vi "KeythleyDMM6500_04582450.vi"(4 "error in":T14, 7 "Command":T15) -> (0 "error out":T14, 3 "Response":T12)   [LabVIEW 2018]
uses:
  MOKO_LabViewLibrary/MokoLowLevel/MokoLowLovelControl/MLLC_Command.ctl
  MOKO_LabViewLibrary/MokoLowLevel/MokoLowLovelControl/MLLC_Error.ctl
  MOKO_LabViewLibrary/MokoLowLevel/MokoLowLovelControl/MLLC_Mode.ctl
  MOKO_LabViewLibrary/MokoLowLevel/MokoLowLovelControl/MLLC_Response.ctl
  MOKO_LabViewLibrary/MokoLowLevel/MokoLowLovelControl/MLLC_DriverName.ctl
  MOKO_LabViewLibrary/MokoLowLevel/MokoLowLovelControl/MLLC_Request.ctl
  MOKO_LabViewLibrary/MokoLowLevel/MokoLowLovelControl/MLLC_ErrorCode.ctl
  MOKO_LabViewLibrary/MokoLowLevel/MokoLowLovelControl/MLLC_ResponseInit.ctl
  MOKO_LabViewLibrary/MokoLowLevel/MokoLowLovelControl/MLLC_ConnectCluster.ctl
  MOKO_LabViewLibrary/MokoLowLevel/MokoLowLovelControl/MLLC_InterfaceType.ctl
  MOKO_LabViewLibrary/MokoLowLevel/MokoLowLovelControl/MLLC_OpenedSession.ctl
  MOKO_LabViewLibrary/MokoLowLevel/MokoLowLovelControl/MLLC_InterfaceSettings.ctl
  MOKO_LabViewLibrary/MokoLowLevel/MokoLowLovelControl/MLLC_InterfaceKind.ctl
  data/KeythleyDMM6500_Functions.ctl
panel:
  in  "Settings":T8={"Saved Data"=variant, "Data"={"Connect"={"InterfaceType"=enum."VISA", "OpenedSession"="", "InterfaceSettings"={"Interface"=enum."GPIB", "EOS 4 read"=enum."LF (\\n)", "EOS 4 write"=enum."LF (\\n)", "TMO, ms"=5000, "Sett"=variant(cluster{"Baud Rate":u32, "Data Bits":u16, "Parity":u16, "Stop Bits":u16, "Flow Control":u16, "Eho":bool} {"Baud Rate"=75, "Data Bits"=0, "Parity"=0, "Stop Bits"=0, "Flow Control"=0, "Eho"=FALSE})}}, "Channel"=1, "Func"=enum."IDC"}}
  in  "Response Init array":T9="DMM6500,04582450"
  in  "Error Code":T6=5475
  in  "Request":T10="*idn?"
  in  "Driver Name":T11="DMM6500_04582450"
  in  "Mode":T13=enum."Check"
  # "KEITHLEY INSTRUMENTS,MODEL DMM6500,04582450,1.7.12b = U"
  # "KEITHLEY INSTRUMENTS,MODEL DMM6500,04625545,1.7.12b = I"
  # "KeythleyDMM6500_04582450"
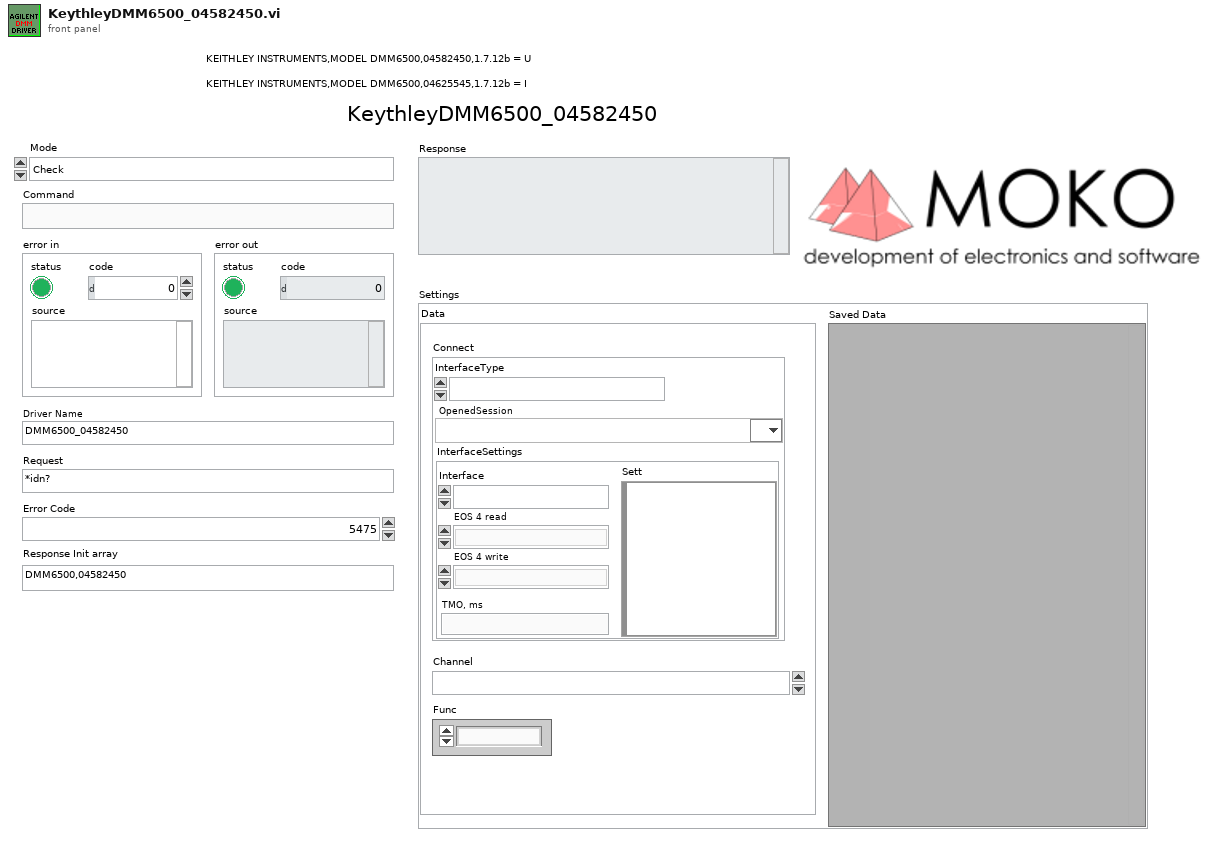
[diagram p1: front panel]
types:
  T1 = typedef "MLLC_ConnectCluster.ctl" = cluster{"InterfaceType":T2, "OpenedSession":T3, "InterfaceSettings":T4}
  T2 = typedef "MLLC_InterfaceType.ctl" = enum16{"VISA", "Prologix USB-GPIB"}
  T3 = typedef "MLLC_OpenedSession.ctl" = refnum<visa-resource-name>
  T4 = typedef "MLLC_InterfaceSettings.ctl" = cluster{"Interface":T5, "EOS 4 read":enum16{"Default (=EOS 4 write)", "CR (\\r)", "LF (\\n)", "None"}, "EOS 4 write":enum16{"CR+LF (\\r\\n)", "CR (\\r)", "LF (\\n)", "None"}, "TMO, ms":i32, "Sett":variant}
  T5 = typedef "MLLC_InterfaceKind.ctl" = enum16{"RS232", "GPIB", "USB", "Ethernet", "another"}
  T6 = typedef "MLLC_ErrorCode.ctl" = u32
  T7 = typedef "KeythleyDMM6500_Functions.ctl" = enum16{"VDC", "VAC", "IDC", "IAC", "F", "R2", "R4", "CAP"}
  T8 = cluster{"Saved Data":variant, "Data":cluster{"Connect":T1, "Channel":T6, "Func":T7}}
  T9 = typedef "MLLC_ResponseInit.ctl" = string
  T10 = typedef "MLLC_Request.ctl" = string
  T11 = typedef "MLLC_DriverName.ctl" = string
  T12 = typedef "MLLC_Response.ctl" = string
  T13 = typedef "MLLC_Mode.ctl" = enum16{"get", "set", "close", "Init", "Check"}
  T14 = typedef "MLLC_Error.ctl" = errorcluster
  T15 = typedef "MLLC_Command.ctl" = string
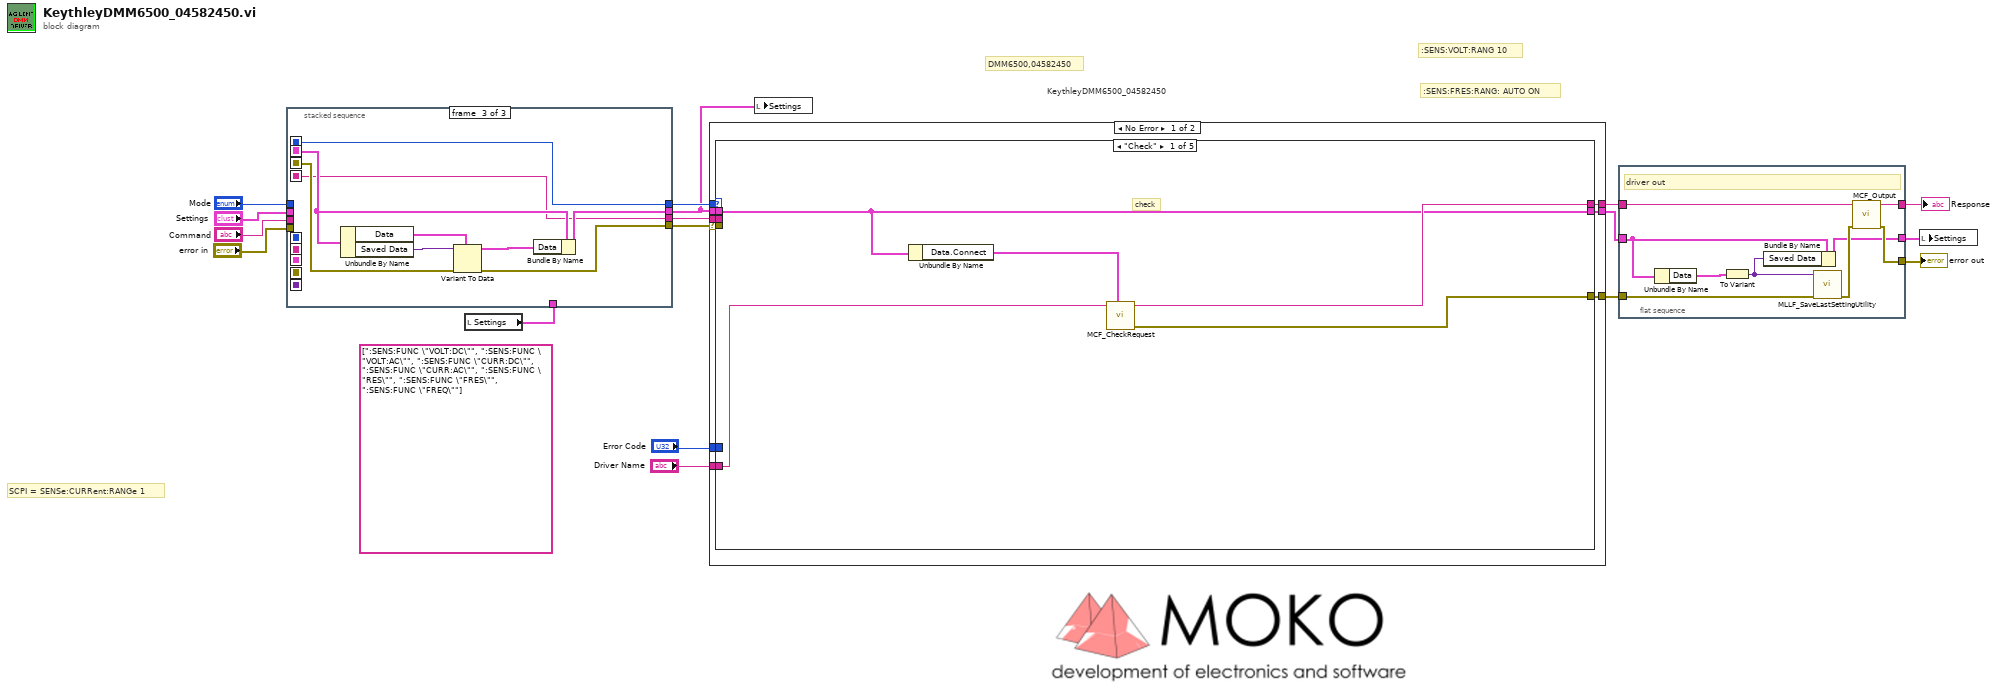
[diagram p0: block diagram]
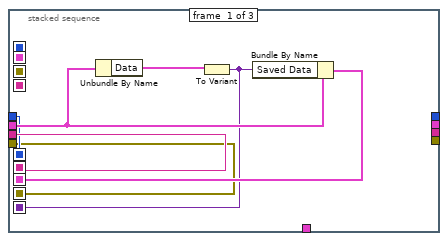
[diagram p2: hidden frame]
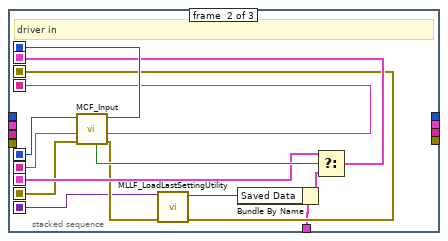
[diagram p3: hidden frame]
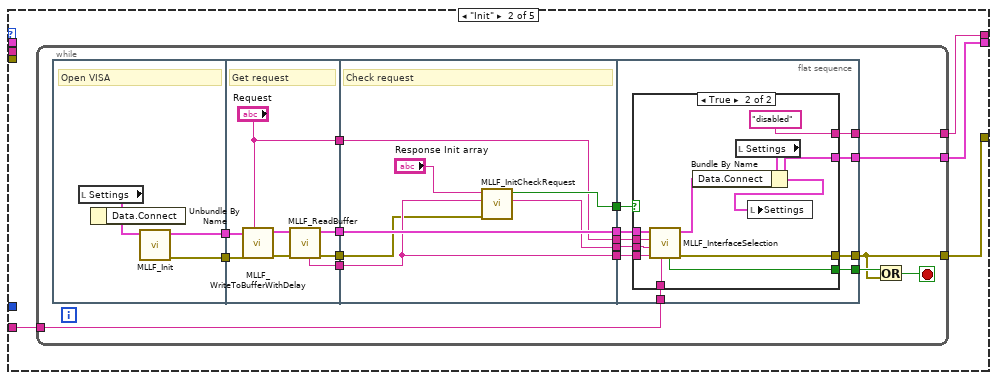
[diagram p4: hidden frame]
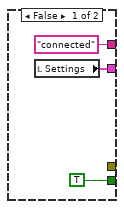
[diagram p5: hidden frame]
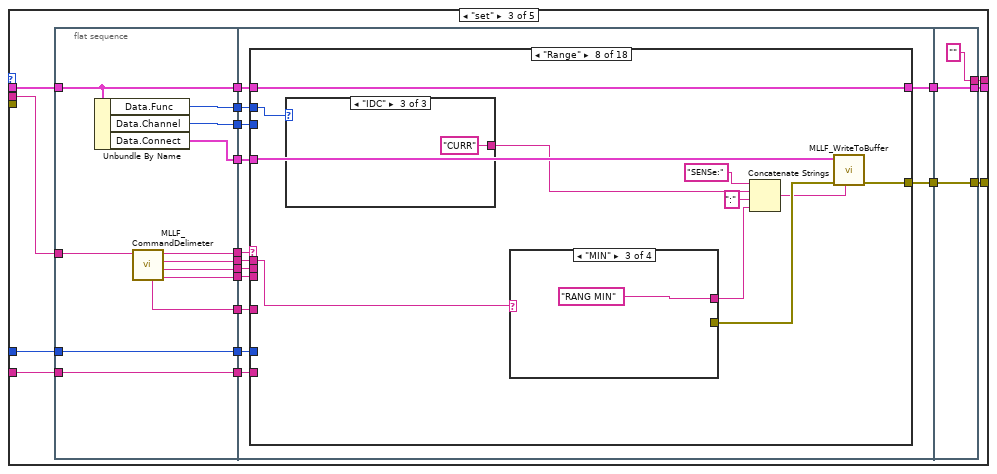
[diagram p6: hidden frame]
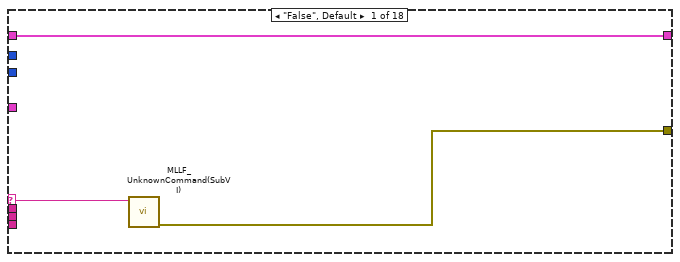
[diagram p7: hidden frame]
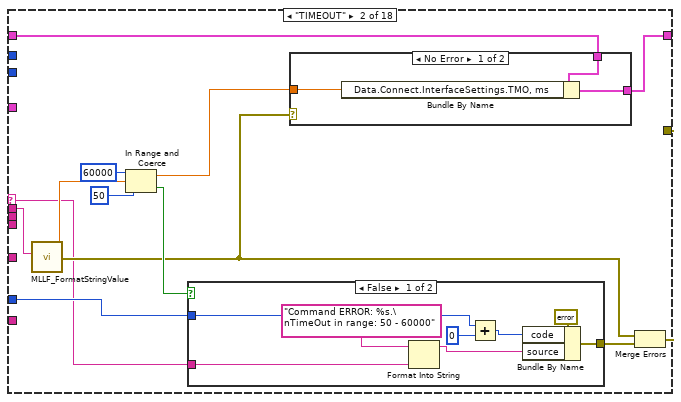
[diagram p8: hidden frame]
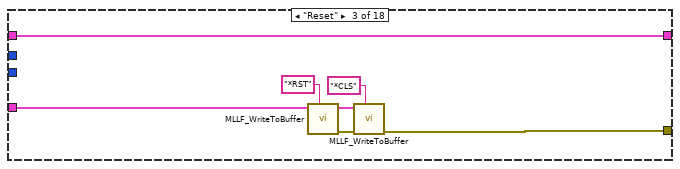
[diagram p11: hidden frame]
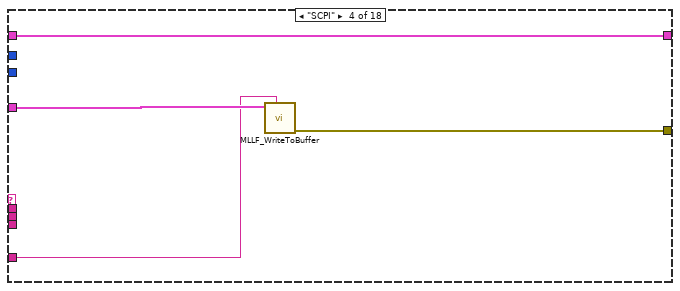
[diagram p12: hidden frame]
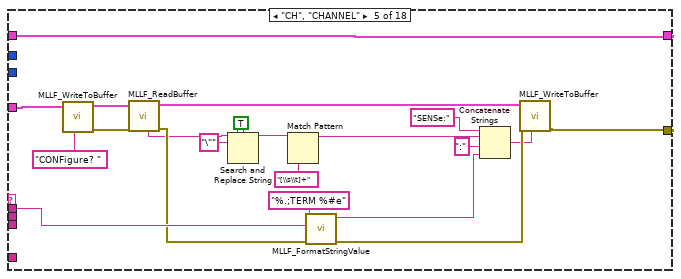
[diagram p13: hidden frame]
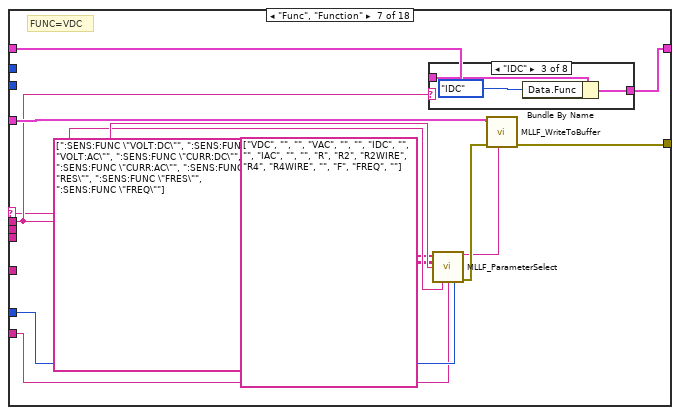
[diagram p15: hidden frame]
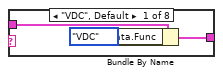
[diagram p16: hidden frame]
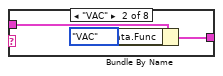
[diagram p17: hidden frame]
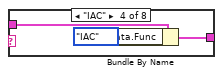
[diagram p18: hidden frame]
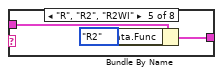
[diagram p19: hidden frame]
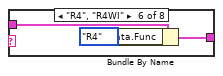
[diagram p20: hidden frame]
diagram:
  (unwired) string[] [":SENS:FUNC \"VOLT:DC\"", ":SENS:FUNC \"VOLT:AC\"", ":SENS:FUNC \"CURR:DC\"", ":SENS:FUNC \"CURR:AC\"", ":SENS:FUNC \"RES\"", ":SENS:FUNC \"FRES\"", ":SENS:FUNC \"FREQ\""] ("Names")
  # ":SENS:FRES:RANG: AUTO ON"
  # ":SENS:VOLT:RANG 10"
  # "DMM6500,04582450"
  # "SCPI = SENSe:CURRent:RANGe 1"
  # "KeythleyDMM6500_04582450"
  n1 = local read "Settings"() -> (w8:T8)
  n2 = stacked-sequence {
    seq-local: [w20 _ _] -> [_ w36 _]
    seq-local: [w19 _ _] -> [_ w37 _]
    seq-local: [w22 _ _] -> [_ w32 _]
    seq-local: [w18 _ _] -> [_ w31 _]
    seq-local: [w21 _ _] -> [_ w27 _]
    seq-local: [_ w28 _] -> [_ _ w44]
    seq-local: [_ w38 _] -> [_ _ w41]
    seq-local: [_ w35 _] -> [_ _ w40]
    seq-local: [_ w34 _] -> [_ _ w45]
    tunnel: "Command" -> [w20 _ _]
    tunnel: "Mode" -> [w19 _ _]
    tunnel: "error in" -> [w18 _ _]
    tunnel: "Settings" -> [w23 _ _]
    tunnel: w8 -> [_ w26 _]
    tunnel: [_ _ w40] -> w10
    tunnel: [_ _ w43] -> w2
    tunnel: [_ _ w42] -> w9
    tunnel: [_ _ w41] -> w11
    frame #0 {
      n3 = Unbundle By Name(w23) -> ("Data"=w24:cluster{"Connect":T1, "Channel":T6, "Func":T7})
      n4 = To Variant(anything=w24) -> (Variant=w21:variant)
      n5 = Bundle By Name(cluster=w23, "Saved Data"=w21) -> (w22:T8)
    }
    frame #1 {
      # "driver in"
      n6 = call "MCF_Input.vi"("Error In"=w31, "Command in"=w36, "Mode in"=w37) -> ("Error Out"=w30:errorcluster, "Command out"=w35:string, "Mode out"=w38:T13, "Boolean"=w33:bool)  [unwired: 5 in]
      n7 = call "MLLF_LoadLastSettingUtility.vi"("Error In"=w30, "Save data in"=w27) -> ("Error Out"=w28:errorcluster, "Save data out"=w25:variant)  [unwired: 8 in]
      n8 = Bundle By Name(cluster=w26, "Saved Data"=w25) -> (w29:T8)
      n9 = Select(t=w32, s=w33, f=w29) -> (s? t:f=w34:T8)
    }
    frame #2 {
      n10 = Unbundle By Name(w45) -> ("Data"=w46:cluster{"Connect":T1, "Channel":T6, "Func":T7}, "Saved Data"=w39:variant)
      n11 = Variant To Data(error in=w44, type=w46, Variant=w39) -> (data=w47:cluster{"Connect":T1, "Channel":T6, "Func":T7}, error out=w42:errorcluster)
      n12 = Bundle By Name(cluster=w45, "Data"=w47) -> (w43:T8)
    }
  }
  n13 = case shown="No Error" w9 {
    selector: w9 -> [w53 w582]
    tunnel: [w54 w582] -> w5
    tunnel: w11 -> [w56 _]
    tunnel: [w55 "An error occurred in the driver input module." ("String")] -> w7
    tunnel: w10 -> [w48 _]
    tunnel: w2 -> [w49 w581]
    tunnel: "Error Code" -> [w52 _]
    tunnel: "Driver Name" -> [w51 _]
    tunnel: [w50 w581] -> w6
    frame No Error {
      n14 = case shown="\"Check\"" w56 {
        tunnel: [w60 w65 w139 w508 "" ("String")] -> w55
        tunnel: [w61 w63 w142 w509 w578] -> w54
        tunnel: w53 -> [_ _ _ w523 _]
        tunnel: w52 -> [_ _ w145 w525 _]
        tunnel: w51 -> [w59 w62 w143 w524 _]
        tunnel: [w57 w64 w144 w526 w577] -> w50
        tunnel: w49 -> [w57 _ w128 w514 w577]
        tunnel: w48 -> [_ _ w127 w513 _]
        frame "Check" {
          # "check"
          n15 = Unbundle By Name(w57) -> ("Data.Connect"=w58:T1)
          n16 = call "MCF_CheckRequest.vi"("Permanent data.Connect"=w58, "Driver Name"=w59) -> ("Error Out"=w61:errorcluster, "Output String"=w60:string)  [unwired: 8 in]
        }
        frame "Init" {
          n17 = while {
            tunnel: [w71] -> w63
            tunnel: [w70] -> w65
            tunnel: [w69] -> w64
            tunnel: w62 -> [w73]
            stop <- w82 stop-if-true
            n18 = flat-sequence {
              tunnel: [w86] -> w81
              tunnel: [w85] -> w80
              tunnel: w81 -> [w92]
              tunnel: w80 -> [w91]
              tunnel: [w90] -> w79
              tunnel: [w89] -> w78
              tunnel: [w88] -> w77
              tunnel: ["Request"] -> w67
              tunnel: w79 -> [w98]
              tunnel: w78 -> [w101]
              tunnel: w77 -> [w100]
              tunnel: [w101] -> w76
              tunnel: [w100] -> w75
              tunnel: [w97] -> w74
              tunnel: [w96] -> w68
              tunnel: w67 -> [w95]
              tunnel: [w95] -> w66
              tunnel: w76 -> [w110]
              tunnel: w75 -> [w109]
              tunnel: w74 -> [w111]
              tunnel: w73 -> [w108]
              tunnel: [w107] -> w72
              tunnel: [w106] -> w71
              tunnel: [w105] -> w70
              tunnel: [w104] -> w69
              tunnel: w68 -> [w103]
              tunnel: w66 -> [w102]
              frame #0 {
                # "Open VISA"
                n19 = local read "Settings"() -> (w84:T8)
                n20 = Unbundle By Name(w84) -> ("Data.Connect"=w83:T1)
                n21 = call "MLLF_Init.vi"("DriverConnect in"=w83) -> ("Error Out"=w86:errorcluster, "DriverConnect out"=w85:T1)  [unwired: 7 in]
              }
              frame #1 {
                # "Get request"
                n22 = call "MLLF_WriteToBufferWithDelay.vi"("Command"="Request", "Error In"=w92, "DriverConnect in"=w91) -> ("Error Out"=w93:errorcluster, "DriverConnect out"=w94:T1)  [unwired: 7 in]
                n23 = call "MLLF_ReadBuffer.vi"("Error In"=w93, "DriverConnect in"=w94) -> ("Error Out"=w90:errorcluster, "DriverConnect out"=w89:T1, "String"=w88:string)  [unwired: 6 in]
              }
              frame #2 {
                # "Check request"
                n24 = call "MLLF_InitCheckRequest.vi"("error in (no error)"=w98, "Answer"=w100, "Response Init"="Response Init array") -> ("ResponseInit out"=w96:string, "Design"=w97:bool)  [unwired: 5 in, 2 out]
              }
              frame #3 {
                n25 = case shown="True" w111 {
                  tunnel: w110 -> [_ w124]
                  tunnel: [TRUE w119] -> w107
                  tunnel: [_ w122] -> w106
                  tunnel: ["connected" "disabled"] -> w105
                  tunnel: [w112 w120] -> w104
                  tunnel: w109 -> [_ w117]
                  tunnel: w108 -> [_ w118]
                  tunnel: w103 -> [_ w116]
                  tunnel: w102 -> [_ w115]
                  frame False {
                    n26 = local read "Settings"() -> (w112:T8)
                  }
                  frame True {
                    n27 = call "MLLF_InterfaceSelection.vi"("Driver Name"=w118, "Answer:"=w117, "Response"=w116, "Request"=w115, "DriverConnect in"=w124) -> ("error out"=w122:T14, "DriverConnect out"=w123:T1, "stop init?"=w119:bool)  [unwired: 2 in, 2 out]
                    n28 = local read "Settings"() -> (w125:T8)
                    n29 = Bundle By Name(cluster=w125, "Data.Connect"=w123) -> (w120:T8)
                    n30 = local write "Settings"(w120) -> ()
                  }
                }
              }
            }
            n31 = Or(x=w72, y=w71) -> (x .or. y?=w82:bool)
          }
        }
        frame "set" {
          n32 = flat-sequence {
            tunnel: w143 -> [w156]
            tunnel: w128 -> [w147]
            tunnel: w145 -> [w157]
            tunnel: [w157] -> w138
            tunnel: [w147] -> w137
            tunnel: [w156] -> w136
            tunnel: [w153] -> w135
            tunnel: [w154] -> w134
            tunnel: [w155] -> w133
            tunnel: [w148] -> w132
            tunnel: [w149] -> w131
            tunnel: [w150] -> w130
            tunnel: [w151] -> w129
            tunnel: w127 -> [w152]
            tunnel: [w146] -> w126
            tunnel: [w168] -> w141
            tunnel: [w161] -> w140
            tunnel: w138 -> [w170]
            tunnel: w137 -> [w169]
            tunnel: w136 -> [w167]
            tunnel: w135 -> [w166]
            tunnel: w134 -> [w165]
            tunnel: w133 -> [w164]
            tunnel: w132 -> [w163]
            tunnel: w131 -> [w162]
            tunnel: w130 -> [w160]
            tunnel: w129 -> [w159]
            tunnel: w126 -> [w158]
            tunnel: [w506] -> w142
            tunnel: [w507] -> w144
            tunnel: w141 -> [w507]
            tunnel: w140 -> [w506]
            tunnel: ["" ("String")] -> w139
            frame #0 {
              n33 = Unbundle By Name(w147) -> ("Data.Func"=w155:T7, "Data.Channel"=w154:T6, "Data.Connect"=w153:T1)
              n34 = call "MLLF_CommandDelimeter.vi"("command with param"=w152) -> ("param 3"=w151:string, "param 2"=w150:string, "param 1"=w149:string, "command"=w148:string, "Spit delimetre"=w146:string)  [unwired: 6 in]
            }
            frame #1 {
              n35 = case shown="\"Range\"" w163 {
                selector: w163 -> [w172 w175 _ _ _ _ w237 _ _ _ _ _ _ w429 w436 w460 w484 w495]
                tunnel: w162 -> [_ w174 _ _ w228 _ w238 w277 _ w307 w320 w361 w391 w430 w437 w461 w485 w496]
                tunnel: [w171 w180 w199 w207 w210 _ w232 w271 _ w290 w319 w345 w376 w409 w435 w459 w483 w494] -> w161
                tunnel: w170 -> [_ w181 _ _ _ _ w243 _ _ _ _ _ _ w431 w441 w465 w489 w503]
                tunnel: w169 -> [w173 w185 w205 w209 w229 w231 w240 w278 w289 w309 w336 w363 w393 w434 w458 w482 w493 w504]
                tunnel: [w173 w186 w205 w209 w229 w231 w239 w278 w289 w309 w336 w363 w393 w434 w458 w482 w493 w504] -> w168
                tunnel: w166 -> [_ _ w200 w208 w230 _ w241 w269 _ w308 w335 w362 w392 w433 w457 w481 w487 w500]
                tunnel: w167 -> [_ _ _ _ _ _ w242 _ _ _ _ _ _ w432 w442 w466 w490 w502]
                tunnel: w165 -> [_ _ _ _ _ _ _ _ _ _ _ _ _ _ _ _ _ _]
                tunnel: w164 -> [_ _ _ _ _ _ _ w270 _ _ _ _ _ _ _ _ _ _]
                tunnel: w160 -> [_ _ _ _ _ _ _ _ _ _ _ _ _ _ _ _ _ _]
                tunnel: w159 -> [_ _ _ _ _ _ _ _ _ _ _ _ _ _ _ _ _ _]
                tunnel: w158 -> [_ _ _ w206 _ _ _ _ _ _ _ _ _ _ _ _ _ _]
                frame "False", Default {
                  n36 = call "MLLF_UnknownCommand(SubVI).vi"("Unknown command"=w172) -> ("error out"=w171:errorcluster)  [unwired: 10 in]
                }
                frame "TIMEOUT" {
                  n37 = call "MLLF_FormatStringValue.vi"("String Value"=w174) -> ("error out"=w176:T14, "number"=w177:dbl)  [unwired: 8 in, 1 out]
                  n38 = In Range and Coerce(upper limit=60000, x=w177, lower limit=50) -> (coerced(x)=w182:dbl, In Range?=w178:bool)
                  n39 = case shown="False" w178 {
                    tunnel: [w193 _] -> w179
                    tunnel: w181 -> [w192 _]
                    tunnel: w175 -> [w191 _]
                    frame False {
                      n40 = Format Into String(format string="Command ERROR: %s.\nTimeOut in range: 50 - 60000", w191) -> (resulting string=w195:string)  [unwired: 2 in, 1 out]
                      n41 = Add(x=w192, y=0) -> (x+y=w196:T6)
                      n42 = Bundle By Name(cluster=errorcluster {"status"=TRUE, "code"=0, "source"=""} ("error out"), "code"=w196, "source"=w195) -> (w193:errorcluster)
                    }
                    frame True {
                    }
                  }
                  n43 = case shown="No Error" w176 {
                    tunnel: [w189 w190] -> w186
                    tunnel: w185 -> [w188 w190]
                    tunnel: w182 -> [w187 _]
                    frame No Error {
                      n44 = Bundle By Name(cluster=w188, "Data.Connect.InterfaceSettings.TMO, ms"=w187) -> (w189:T8)
                    }
                    frame Error {
                    }
                  }
                  n45 = Merge Errors(w176, w179) -> (w180:errorcluster)
                }
                frame "Reset" {
                  n46 = call "MLLF_WriteToBuffer.vi"("String"="*RST", "DriverConnect in"=w200) -> ("error out"=w203:T14, "DriverConnect out"=w204:T1)  [unwired: 6 in]
                  n47 = call "MLLF_WriteToBuffer.vi"("String"="*CLS" ("write buffer"), "error in"=w203, "DriverConnect in"=w204) -> ("error out"=w199:T14)  [unwired: 5 in, 1 out]
                }
                frame "SCPI" {
                  n48 = call "MLLF_WriteToBuffer.vi"("String"=w206, "DriverConnect in"=w208) -> ("error out"=w207:T14)  [unwired: 6 in, 1 out]
                }
                frame "CH", "CHANNEL" {
                  w215 = TRUE ("replace all? (F)")
                  n49 = call "MLLF_WriteToBuffer.vi"("String"="CONFigure? ", "DriverConnect in"=w230) -> ("error out"=w224:T14, "DriverConnect out"=w225:T1)  [unwired: 6 in]
                  n50 = call "MLLF_ReadBuffer.vi"("Error In"=w224, "DriverConnect in"=w225) -> ("Error Out"=w223:errorcluster, "DriverConnect out"=w222:T1, "String"=w217:string)  [unwired: 6 in]
                  n51 = Search and Replace String(replace all?=w215, case sensitive?=w215, input string=w217, search string="\"") -> (result string=w216:string)  [unwired: 4 in, 3 out]
                  n52 = Match Pattern(string=w216, regular expression="[\\s\\t]+") -> (before substring=w218:string)  [unwired: 1 in, 3 out]
                  n53 = call "MLLF_FormatStringValue.vi"("error in"=w223, "String Value"=w228, "Format"="%.;TERM %#e" ("format string")) -> ("error out"=w227:T14, "String Value Formated"=w220:T15)  [unwired: 6 in, 1 out]
                  n54 = Concatenate Strings("SENSe:" ("string"), w218, ":" ("string"), w220) -> (w213:string)
                  n55 = call "MLLF_WriteToBuffer.vi"("String"=w213, "error in"=w227, "DriverConnect in"=w222) -> ("error out"=w210:T14)  [unwired: 5 in, 1 out]
                }
                frame "<----MAIN FUNCTIONS---->" {
                }
                frame "Func", "Function" {
                  # "FUNC=VDC"
                  n56 = case shown="\"IDC\"" w238 {
                    tunnel: w240 -> [w246 w249 w252 w255 w258 w261 w264 w267]
                    tunnel: [w245 w248 w251 w254 w257 w260 w263 w266] -> w239
                    frame "VDC", Default {
                      n57 = Bundle By Name(cluster=w246, "Data.Func"=KeythleyDMM6500_Functions."VDC" ("Func")) -> (w245:T8)
                    }
                    frame "VAC" {
                      n58 = Bundle By Name(cluster=w249, "Data.Func"=KeythleyDMM6500_Functions."VAC" ("Func")) -> (w248:T8)
                    }
                    frame "IDC" {
                      n59 = Bundle By Name(cluster=w252, "Data.Func"=KeythleyDMM6500_Functions."IDC" ("Func")) -> (w251:T8)
                    }
                    frame "IAC" {
                      n60 = Bundle By Name(cluster=w255, "Data.Func"=KeythleyDMM6500_Functions."IAC" ("Func")) -> (w254:T8)
                    }
                    frame "R", "R2", "R2WI" {
                      n61 = Bundle By Name(cluster=w258, "Data.Func"=KeythleyDMM6500_Functions."R2" ("Func")) -> (w257:T8)
                    }
                    frame "R4", "R4WI" {
                      n62 = Bundle By Name(cluster=w261, "Data.Func"=KeythleyDMM6500_Functions."R4" ("Func")) -> (w260:T8)
                    }
                    frame "F" {
                      n63 = Bundle By Name(cluster=w264, "Data.Func"=KeythleyDMM6500_Functions."F" ("Func")) -> (w263:T8)
                    }
                    frame "C", "CAP" {
                      n64 = Bundle By Name(cluster=w267, "Data.Func"=KeythleyDMM6500_Functions."CAP" ("Func")) -> (w266:T8)
                    }
                  }
                  n65 = call "MLLF_ParameterSelect.vi"("Command to equipment"=string[] [":SENS:FUNC \"VOLT:DC\"", ":SENS:FUNC \"VOLT:AC\"", ":SENS:FUNC \"CURR:DC\"", ":SENS:FUNC \"CURR:AC\"", ":SENS:FUNC \"RES\"", ":SENS:FUNC \"FRES\"", ":SENS:FUNC \"FREQ\""] ("Names"), "Names"=string[][] [["VDC", "", ""], ["VAC", "", ""], ["IDC", "", ""], ["IAC", "", ""], ["R", "R2", "R2WIRE"], ["R4", "R4WIRE", ""], ["F", "FREQ", ""]], "Input"=w238, "Command"=w237, "Driver Name"=w242, "Error Code"=w243) -> ("Choice"=w233:string, "Error Out"=w234:errorcluster)  [unwired: 8 in]
                  n66 = call "MLLF_WriteToBuffer.vi"("String"=w233, "error in"=w234, "DriverConnect in"=w241) -> ("error out"=w232:T14)  [unwired: 5 in, 1 out]
                }
                frame "Range" {
                  n67 = case shown="\"IDC\"" w270 {
                    tunnel: ["VOLT" ("String") "VOLT:AC" ("String") "CURR" ("String")] -> w268
                    frame "VDC", Default {
                    }
                    frame "VAC" {
                    }
                    frame "IDC" {
                    }
                  }
                  n68 = case shown="\"MIN\"" w277 {
                    selector: w277 -> [w282 _ _ _]
                    tunnel: [w285 _ _ _] -> w276
                    tunnel: [w284 "RANG:AUTO ON" ("String") "RANG MIN" ("String") "RANG MAX" ("String")] -> w275
                    frame "False", Default {
                      n69 = call "MLLF_FormatStringValue.vi"("String Value"=w282, "Format"="RANG %#e" ("format string")) -> ("error out"=w285:T14, "String Value Formated"=w284:T15)  [unwired: 7 in, 1 out]
                    }
                    frame "Auto" {
                    }
                    frame "MIN" {
                    }
                    frame "MAX" {
                    }
                  }
                  n70 = Concatenate Strings("SENSe:" ("string"), w268, ":" ("string"), w275) -> (w273:string)
                  n71 = call "MLLF_WriteToBuffer.vi"("String"=w273, "error in"=w276, "DriverConnect in"=w269) -> ("error out"=w271:T14)  [unwired: 5 in, 1 out]
                }
                frame "---------ADDITIONAL---------" {
                }
                frame "Res", "Resolution" {
                  w294 = TRUE ("replace all? (F)")
                  n72 = call "MLLF_WriteToBuffer.vi"("String"="CONFigure? ", "DriverConnect in"=w308) -> ("error out"=w303:T14, "DriverConnect out"=w304:T1)  [unwired: 6 in]
                  n73 = call "MLLF_ReadBuffer.vi"("Error In"=w303, "DriverConnect in"=w304) -> ("Error Out"=w302:errorcluster, "DriverConnect out"=w301:T1, "String"=w296:string)  [unwired: 6 in]
                  n74 = Search and Replace String(replace all?=w294, case sensitive?=w294, input string=w296, search string="\"") -> (result string=w295:string)  [unwired: 4 in, 3 out]
                  n75 = case shown="\"MIN\"" w307 {
                    selector: w307 -> [w311 _ _]
                    tunnel: [w314 w315 w317] -> w306
                    tunnel: [w313 "RES MAX" ("String") "RES MIN" ("String")] -> w299
                    tunnel: w302 -> [w310 w315 w317]
                    frame "False", Default {
                      n76 = call "MLLF_FormatStringValue.vi"("error in"=w310, "String Value"=w311, "Format"="RES %#e" ("format string")) -> ("error out"=w314:T14, "String Value Formated"=w313:T15)  [unwired: 6 in, 1 out]
                    }
                    frame "MAX" {
                    }
                    frame "MIN" {
                    }
                  }
                  n77 = Match Pattern(string=w295, regular expression="[\\s\\t]+") -> (before substring=w297:string)  [unwired: 1 in, 3 out]
                  n78 = Concatenate Strings("SENSe:" ("string"), w297, ":" ("string"), w299) -> (w292:string)
                  n79 = call "MLLF_WriteToBuffer.vi"("String"=w292, "error in"=w306, "DriverConnect in"=w301) -> ("error out"=w290:T14)  [unwired: 5 in, 1 out]
                }
                frame "Aper", "Aperture", "MeasTime" {
                  w323 = TRUE ("replace all? (F)")
                  n80 = call "MLLF_WriteToBuffer.vi"("String"="CONFigure? ", "DriverConnect in"=w335) -> ("error out"=w332:T14, "DriverConnect out"=w333:T1)  [unwired: 6 in]
                  n81 = call "MLLF_ReadBuffer.vi"("Error In"=w332, "DriverConnect in"=w333) -> ("Error Out"=w331:errorcluster, "DriverConnect out"=w330:T1, "String"=w325:string)  [unwired: 6 in]
                  n82 = Search and Replace String(replace all?=w323, case sensitive?=w323, input string=w325, search string="\"") -> (result string=w324:string)  [unwired: 4 in, 3 out]
                  n83 = case shown="\"OFF\"" w320 {
                    selector: w320 -> [w339 _]
                    tunnel: [w342 w343] -> w337
                    tunnel: [w341 "APER:ENAB OFF" ("String")] -> w328
                    tunnel: w331 -> [w338 w343]
                    frame "False", Default {
                      n84 = call "MLLF_FormatStringValue.vi"("error in"=w338, "String Value"=w339, "Format"="APER %#e" ("format string")) -> ("error out"=w342:T14, "String Value Formated"=w341:T15)  [unwired: 6 in, 1 out]
                    }
                    frame "OFF" {
                    }
                  }
                  n85 = Match Pattern(string=w324, regular expression="[\\s\\t]+") -> (before substring=w326:string)  [unwired: 1 in, 3 out]
                  n86 = Concatenate Strings(w326, ":" ("string"), w328) -> (w321:string)
                  n87 = call "MLLF_WriteToBuffer.vi"("String"=w321, "error in"=w337, "DriverConnect in"=w330) -> ("error out"=w319:T14)  [unwired: 5 in, 1 out]
                }
                frame "IntegrationTime", "IntTime", "NPLC" {
                  w349 = TRUE ("replace all? (F)")
                  n88 = call "MLLF_WriteToBuffer.vi"("String"="CONFigure? ", "DriverConnect in"=w362) -> ("error out"=w357:T14, "DriverConnect out"=w358:T1)  [unwired: 6 in]
                  n89 = call "MLLF_ReadBuffer.vi"("Error In"=w357, "DriverConnect in"=w358) -> ("DriverConnect out"=w356:T1, "String"=w351:string)  [unwired: 6 in, 1 out]
                  n90 = Search and Replace String(replace all?=w349, case sensitive?=w349, input string=w351, search string="\"") -> (result string=w350:string)  [unwired: 4 in, 3 out]
                  n91 = case shown="\"MIN\"" w361 {
                    tunnel: [w367 w371 w375] -> w360
                    tunnel: [w366 w370 w374] -> w354
                    tunnel: w361 -> [w364 w368 w372]
                    frame Default {
                      n92 = call "MLLF_FormatStringValue.vi"("String Value"=w364, "Format"="NPLC %#e" ("format string")) -> ("error out"=w367:T14, "String Value Formated"=w366:T15)  [unwired: 7 in, 1 out]
                    }
                    frame "MIN" {
                      n93 = call "MLLF_FormatStringValue.vi"("String Value"=w368, "Format"="NPLC MIN" ("format string")) -> ("error out"=w371:T14, "String Value Formated"=w370:T15)  [unwired: 7 in, 1 out]
                    }
                    frame "MAX" {
                      n94 = call "MLLF_FormatStringValue.vi"("String Value"=w372, "Format"="NPLC MAX" ("format string")) -> ("error out"=w375:T14, "String Value Formated"=w374:T15)  [unwired: 7 in, 1 out]
                    }
                  }
                  n95 = Match Pattern(string=w350, regular expression="[\\s\\t]+") -> (before substring=w352:string)  [unwired: 1 in, 3 out]
                  n96 = Concatenate Strings("SENSe:" ("string"), w352, ":" ("string"), w354) -> (w347:string)
                  n97 = call "MLLF_WriteToBuffer.vi"("String"=w347, "error in"=w360, "DriverConnect in"=w356) -> ("error out"=w345:T14)  [unwired: 5 in, 1 out]
                }
                frame "ACBand", "ACBandwidth", "Band", "Bandwidth" {
                  w380 = TRUE ("replace all? (F)")
                  n98 = call "MLLF_WriteToBuffer.vi"("String"="CONFigure? ", "DriverConnect in"=w392) -> ("error out"=w387:T14, "DriverConnect out"=w388:T1)  [unwired: 6 in]
                  n99 = call "MLLF_ReadBuffer.vi"("Error In"=w387, "DriverConnect in"=w388) -> ("Error Out"=w386:errorcluster, "DriverConnect out"=w385:T1, "String"=w382:string)  [unwired: 6 in]
                  n100 = case shown="\"MAX\"" w391 {
                    tunnel: [w398 w403 w408] -> w390
                    tunnel: w386 -> [w397 w402 w407]
                    tunnel: [w396 w401 w406] -> w383
                    tunnel: w391 -> [w394 w399 w404]
                    frame Default {
                      n101 = call "MLLF_FormatStringValue.vi"("error in"=w397, "String Value"=w394, "Format"="BAND %#f" ("format string")) -> ("error out"=w398:T14, "String Value Formated"=w396:T15)  [unwired: 6 in, 1 out]
                    }
                    frame "MAX" {
                      n102 = call "MLLF_FormatStringValue.vi"("error in"=w402, "String Value"=w399, "Format"="BAND MAX" ("format string")) -> ("error out"=w403:T14, "String Value Formated"=w401:T15)  [unwired: 6 in, 1 out]
                    }
                    frame "MIN" {
                      n103 = call "MLLF_FormatStringValue.vi"("error in"=w407, "String Value"=w404, "Format"="BAND MIN" ("format string")) -> ("error out"=w408:T14, "String Value Formated"=w406:T15)  [unwired: 6 in, 1 out]
                    }
                  }
                  n104 = Search and Replace String(replace all?=w380, case sensitive?=w380, input string=w382, search string="\"") -> (result string=w381:string)  [unwired: 4 in, 3 out]
                  n105 = Match Pattern(string=w381, regular expression="[\\s\\t]+") -> ()  [unwired: 1 in, 4 out]
                  n106 = Concatenate Strings(":DET:" ("string"), w383) -> (w378:string)
                  n107 = call "MLLF_WriteToBuffer.vi"("String"=w378, "error in"=w390, "DriverConnect in"=w385) -> ("error out"=w376:T14)  [unwired: 5 in, 1 out]
                }
                frame "AutoZero", "ZERO" {
                  w419 = TRUE ("replace all? (F)")
                  n108 = call "MLLF_WriteToBuffer.vi"("String"="CONFigure? ", "DriverConnect in"=w433) -> ("error out"=w426:T14, "DriverConnect out"=w427:T1)  [unwired: 6 in]
                  n109 = call "MLLF_ReadBuffer.vi"("Error In"=w426, "DriverConnect in"=w427) -> ("Error Out"=w413:errorcluster, "DriverConnect out"=w425:T1, "String"=w421:string)  [unwired: 6 in]
                  n110 = Search and Replace String(replace all?=w419, case sensitive?=w419, input string=w421, search string="\"") -> (result string=w420:string)  [unwired: 4 in, 3 out]
                  n111 = Match Pattern(string=w420, regular expression="[\\s\\t]+") -> (before substring=w422:string)  [unwired: 1 in, 3 out]
                  n112 = call "MLLF_ParameterSelect.vi"("Command to equipment"=string[] ["ZERO:AUTO OFF", "ZERO:AUTO ON", "ZERO:AUTO ONCE"] ("Names"), "Ignor case(default = true)"=TRUE, "Names"=string[][] [["OFF"], ["ON"], ["ONCE"]], "Input"=w430, "Error In"=w413, "Command"=w429, "Driver Name"=w432, "Error Code"=w431) -> ("Choice"=w412:string, "Error Out"=w414:errorcluster)  [unwired: 6 in]
                  n113 = Concatenate Strings("SENSe:" ("string"), w422, ":" ("string"), w412) -> (w417:string)
                  n114 = call "MLLF_WriteToBuffer.vi"("String"=w417, "error in"=w414, "DriverConnect in"=w425) -> ("error out"=w409:T14)  [unwired: 5 in, 1 out]
                }
                frame "LOWPOWER" {
                  w447 = TRUE ("replace all? (F)")
                  n115 = call "MLLF_WriteToBuffer.vi"("String"="CONFigure? ", "DriverConnect in"=w457) -> ("error out"=w454:T14, "DriverConnect out"=w455:T1)  [unwired: 6 in]
                  n116 = call "MLLF_ReadBuffer.vi"("Error In"=w454, "DriverConnect in"=w455) -> ("Error Out"=w439:errorcluster, "DriverConnect out"=w453:T1, "String"=w449:string)  [unwired: 6 in]
                  n117 = Search and Replace String(replace all?=w447, case sensitive?=w447, input string=w449, search string="\"") -> (result string=w448:string)  [unwired: 4 in, 3 out]
                  n118 = Match Pattern(string=w448, regular expression="[\\s\\t]+") -> (before substring=w450:string)  [unwired: 1 in, 3 out]
                  n119 = call "MLLF_ParameterSelect.vi"("Command to equipment"=string[] ["POW:LIM OFF", "POW:LIM ON"] ("Names"), "Names"=string[][] [["0", "DIS", "DISABLE", "DISABLED", "OFF"], ["1", "EN", "ENABLE", "ENABLED", "ON"]], "Input"=w437, "Error In"=w439, "Command"=w436, "Driver Name"=w442, "Error Code"=w441) -> ("Choice"=w438:string, "Error Out"=w440:errorcluster)  [unwired: 7 in]
                  n120 = Concatenate Strings(w450, ":" ("string"), w438) -> (w445:string)
                  n121 = call "MLLF_WriteToBuffer.vi"("String"=w445, "error in"=w440, "DriverConnect in"=w453) -> ("error out"=w435:T14)  [unwired: 5 in, 1 out]
                }
                frame "VOLTAGELIMITED" {
                  w471 = TRUE ("replace all? (F)")
                  n122 = call "MLLF_WriteToBuffer.vi"("String"="CONFigure? ", "DriverConnect in"=w481) -> ("error out"=w478:T14, "DriverConnect out"=w479:T1)  [unwired: 6 in]
                  n123 = call "MLLF_ReadBuffer.vi"("Error In"=w478, "DriverConnect in"=w479) -> ("Error Out"=w463:errorcluster, "DriverConnect out"=w477:T1, "String"=w473:string)  [unwired: 6 in]
                  n124 = Search and Replace String(replace all?=w471, case sensitive?=w471, input string=w473, search string="\"") -> (result string=w472:string)  [unwired: 4 in, 3 out]
                  n125 = Match Pattern(string=w472, regular expression="[\\s\\t]+") -> (before substring=w474:string)  [unwired: 1 in, 3 out]
                  n126 = call "MLLF_ParameterSelect.vi"("Command to equipment"=string[] ["VOLT:LIM OFF", "VOLT:LIM ON"] ("Names"), "Names"=string[][] [["0", "DIS", "DISABLE", "DISABLED", "OFF"], ["1", "EN", "ENABLE", "ENABLED", "ON"]], "Input"=w461, "Error In"=w463, "Command"=w460, "Driver Name"=w466, "Error Code"=w465) -> ("Choice"=w462:string, "Error Out"=w464:errorcluster)  [unwired: 7 in]
                  n127 = Concatenate Strings(w474, ":" ("string"), w462) -> (w469:string)
                  n128 = call "MLLF_WriteToBuffer.vi"("String"=w469, "error in"=w464, "DriverConnect in"=w477) -> ("error out"=w459:T14)  [unwired: 5 in, 1 out]
                }
                frame "FILT", "FILTER" {
                  # "FILT=DIS"
                  n129 = call "MLLF_ParameterSelect.vi"("Command to equipment"=string[] ["INPut:FILTer:STATE OFF", "INPut:FILTer:STATE ON"] ("Names"), "Names"=string[][] [["0", "DIS", "DISABLE", "DISABLED", "OFF"], ["1", "EN", "ENABLE", "ENABLED", "ON"]], "Input"=w485, "Command"=w484, "Driver Name"=w490, "Error Code"=w489) -> ("Choice"=w486:string, "Error Out"=w488:errorcluster)  [unwired: 8 in]
                  n130 = call "MLLF_WriteToBuffer.vi"("String"=w486, "error in"=w488, "DriverConnect in"=w487) -> ("error out"=w483:T14)  [unwired: 5 in, 1 out]
                }
                frame "SND", "Sound" {
                  # "sound"
                  # "sound=off"
                  n131 = call "MLLF_ParameterSelect.vi"("Command to equipment"=string[] ["SYST:BEEP:STAT OFF", "SYST:BEEP:STAT ON", "SYST:BEEP"] ("Names"), "Names"=string[][] [["0", "DIS", "DISABLED", "DISABLE", "OFF"], ["1", "EN", "ENABLE", "ENABLED", "ON"], [" ", "", "", "", ""]], "Input"=w496, "Command"=w495, "Driver Name"=w502, "Error Code"=w503) -> ("Choice"=w499:string, "Error Out"=w501:errorcluster)  [unwired: 8 in]
                  n132 = call "MLLF_WriteToBuffer.vi"("String"=w499, "error in"=w501, "DriverConnect in"=w500) -> ("error out"=w494:T14)  [unwired: 5 in, 1 out]
                }
              }
            }
            frame #2 {
            }
          }
        }
        frame "get" {
          n133 = flat-sequence {
            tunnel: w523 -> [w533]
            tunnel: w524 -> [w534]
            tunnel: w525 -> [w535]
            tunnel: w514 -> [w528]
            tunnel: [w528] -> w522
            tunnel: [w535] -> w521
            tunnel: [w534] -> w520
            tunnel: [w532] -> w519
            tunnel: [w531] -> w518
            tunnel: [w529] -> w517
            tunnel: [w527] -> w516
            tunnel: [w533] -> w515
            tunnel: w513 -> [w530]
            tunnel: w522 -> [w546]
            tunnel: w521 -> [w544]
            tunnel: w520 -> [w543]
            tunnel: w519 -> [w541]
            tunnel: w518 -> [w540]
            tunnel: w517 -> [w539]
            tunnel: w516 -> [w538]
            tunnel: w515 -> [w536]
            tunnel: [w545] -> w512
            tunnel: [w542] -> w511
            tunnel: [w537] -> w510
            tunnel: [w575] -> w526
            tunnel: w512 -> [w575]
            tunnel: w511 -> [w574]
            tunnel: w510 -> [w573]
            tunnel: [w574] -> w509
            tunnel: [w573] -> w508
            frame #0 {
              n134 = Unbundle By Name(w528) -> ("Data.Connect"=w532:T1, "Data.Func"=w531:T7)
              n135 = call "MLLF_CommandDelimeter.vi"("command with param"=w530) -> ("command"=w529:string, "Spit delimetre"=w527:string)  [unwired: 6 in, 3 out]
            }
            frame #1 {
              n136 = case shown="\"READ\"" w539 {
                selector: w539 -> [w548 _ _ _]
                tunnel: [w547 w552 w555 w566] -> w542
                tunnel: w544 -> [_ _ _ _]
                tunnel: [w549 w553 w564 w572] -> w545
                tunnel: w546 -> [w549 w553 w564 w572]
                tunnel: w541 -> [_ _ w563 w571]
                tunnel: w543 -> [_ _ _ _]
                tunnel: w538 -> [_ _ _ w568]
                tunnel: w540 -> [_ _ _ _]
                tunnel: [_ w550 w556 w567] -> w537
                tunnel: w536 -> [_ w552 _ _]
                frame "False", Default {
                  n137 = call "MLLF_UnknownCommand(SubVI).vi"("Unknown command"=w548) -> ("error out"=w547:errorcluster)  [unwired: 10 in]
                }
                frame "TIMEOUT" {
                  n138 = Unbundle By Name(w553) -> ("Data.Connect.InterfaceSettings.TMO, ms"=w551:i32)
                  n139 = Format Value(value (0)=w551) -> (output string=w550:string)  [unwired: 2 in]
                }
                frame "READ" {
                  n140 = call "MLLF_WriteToBufferWithDelay.vi"("Delay Time ( 0,05 s)"=0.05 ("Delay Time (s)"), "Command"="READ?" ("String"), "DriverConnect in"=w563) -> ("Error Out"=w562:errorcluster, "DriverConnect out"=w561:T1)  [unwired: 7 in]
                  n141 = call "MLLF_ReadBuffer.vi"("Error In"=w562, "DriverConnect in"=w561) -> ("Error Out"=w555:errorcluster, "String"=w558:string)  [unwired: 6 in, 1 out]
                  n142 = Fract/Exp String To Number(use system decimal point (T)=FALSE, string=w558) -> (number=w557:dbl)  [unwired: 2 in, 1 out]
                  n143 = Format Value(value (0)=w557) -> (output string=w556:string)  [unwired: 2 in]
                }
                frame "SCPI" {
                  n144 = call "MLLF_WriteToBufferWithDelay.vi"("Delay Time ( 0,05 s)"=0.05 ("Delay Time (s)"), "Command"=w568, "DriverConnect in"=w571) -> ("Error Out"=w570:errorcluster, "DriverConnect out"=w569:T1)  [unwired: 7 in]
                  n145 = call "MLLF_ReadBuffer.vi"("Error In"=w570, "DriverConnect in"=w569) -> ("Error Out"=w566:errorcluster, "String"=w567:string)  [unwired: 6 in, 1 out]
                }
              }
            }
            frame #2 {
            }
          }
        }
        frame "close" {
          n146 = Unbundle By Name(w577) -> ("Data.Connect.OpenedSession"=w579:T3)
          n147 = VISA Close(VISA resource name=w579) -> (error out=w578:errorcluster)  [unwired: 1 in]
        }
      }
    }
    frame Error {
    }
  }
  n148 = local write "Settings"(w2) -> ()
  n149 = flat-sequence {
    tunnel: [w591] -> w1
    tunnel: [w590] -> w4
    tunnel: w7 -> [w589]
    tunnel: w5 -> [w588]
    tunnel: w6 -> [w584]
    tunnel: [w586] -> w3
    frame #0 {
      # "driver out"
      n150 = Unbundle By Name(w584) -> ("Data"=w583:cluster{"Connect":T1, "Channel":T6, "Func":T7})
      n151 = To Variant(anything=w583) -> (Variant=w585:variant)
      n152 = Bundle By Name(cluster=w584, "Saved Data"=w585) -> (w586:T8)
      n153 = call "MLLF_SaveLastSettingUtility.vi"("error in"=w588, "Saved Data"=w585) -> ("error out"=w587:T14)  [unwired: 8 in, 1 out]
      n154 = call "MCF_Output.vi"("Error In"=w587, "Input"=w589) -> ("Error Out"=w590:errorcluster, "Output"=w591:string)  [unwired: 8 in]
    }
  }
  n155 = local write "Settings"(w3) -> ()
  "error out" <- w4
  "Response" <- w1
